vi "ex_setListBoxColumnWidths.vi"(1 "table data":string[][](array[string]), 2 "MCListbox Refnum":refnum<vi>) -> ()   [LabVIEW 2017]
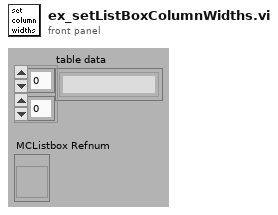
[diagram p1: front panel]
types:
  T1 = enum16{"User-specified Font", "Application Font", "System Font", "Dialog Font"}
  T2 = cluster{"left":i16, "top":i16, "right":i16, "bottom":i16}
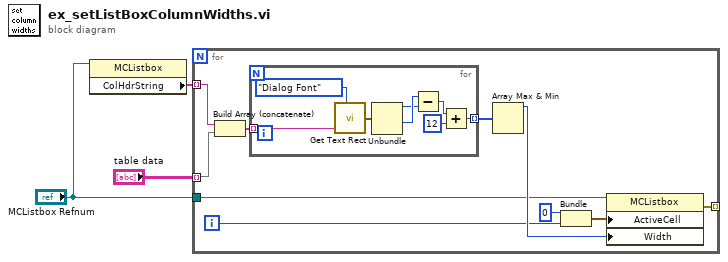
[diagram p0: block diagram]
diagram:
  n1 = property on="Property Node" class="MCListbox"(reference="MCListbox Refnum") -> ("ColHdrString"=w1:string[])  [unwired: 1 in, 2 out]
  n2 = for {
    tunnel: "table data" -> [w6] mode=indexing
    tunnel: "MCListbox Refnum" -> [w8]
    tunnel: w1 -> [w7] mode=indexing
    tunnel: [w4] -> _ mode=indexing
    i -> [w9]
    n3 = Build Array (concatenate)(w7, w6) -> (w5:string[])
    n4 = for {
      tunnel: [w16] -> w12 mode=indexing
      tunnel: w5 -> [w14] mode=indexing
      n5 = call <vilib>:"Get Text Rect.vi"("desired font(Application)"=T1."Dialog Font", "text"=w14) -> ("rect"=w21:T2)  [unwired: 4 in, 3 out]
      n6 = Unbundle(w21) -> ("left"=w19:i16, "right"=w20:i16)  [unwired: 2 out]
      n7 = Subtract(x=w20, y=w19) -> (x-y=w18:i16)
      n8 = Add(x=w18, y=i16 12) -> (x+y=w16:i16)
    }
    n9 = Array Max & Min(array=w12) -> (max value=w11:i16)  [unwired: 3 out]
    n10 = Bundle(0, w9) -> (w13:cluster{i32, i32})  [unwired: 1 out]
    n11 = property on="Property Node" class="MCListbox"(reference=w8, "ActiveCell"=w13, "Width"=w11) -> (error out=w4:errorcluster)  [unwired: 1 in, 1 out]
  }
